vi "fill_sens_dat.vi"(6 "f_temp":T5 format="%_4g", 7 "rh_0":T1 caption="Relative Humidity (%)" format="%#_4g", 9 "raw_dat":string, 10 "index":i32, 11 "element in":T2={"states"=enum."idle", "bytes read"=0, "Response"="", "wr_buffr"="", "bytes_at_port"=0, "temp_clstr"={"sen_4_num"=0.0, "sen_3_num"=0.0, "sen_2_num"=0.0, "sen_1_num"=0.0, "sen_8_num"=0.0, "sen_7_num"=0.0, "sen_6_num"=0.0, "sen_5_num"=0.0, "dts"="", "sen_4"="", "sen_3"="", "sen_2"="", "sen_1"="", "sen_8"="", "sen_7"="", "sen_6"="", "sen_5"="", "temp_f_arry"=[], "sens_dat_raw_arry"=[], "raw_dat"="", "rh_arry"=[], "rh_1"=0.0, "rh_0"=0.0, "rh_3"=0.0, "rh_2"=0.0, "rh_5"=0.0, "rh_4"=0.0, "rh_7"=0.0, "rh_6"=0.0}, "logTable in"=[[["", "", "", "", "", "", "", "", "", ""], ["", "", "", "", "", "", "", "", "", ""], ["", "", "", "", "", "", "", "", "", ""], ["", "", "", "", "", "", "", "", "", ""], ["", "", "", "", "", "", "", "", "", ""], ["", "", "", "", "", "", "", "", "", ""], ["", "", "", "", "", "", "", "", "", " "]]], "mult_list"=0, "log_tabl_row_cnt"=0, "above_row_7"=FALSE, "sens_type"=0, "sens_type_arry"=[], "pibs_clstr"={"sens_typ_str"="", "rh_1"=0.0, "sen_8"="", "sen_7"="", "sen_6"="", "sen_5"="", "sen_4"="", "sen_3"="", "sen_2"="", "sen_1_num"=0.0, "sen_1"="", "rh_2"=0.0, "rh_3"=0.0, "sen_2_num"=0.0, "sen_3_num"=0.0, "sen_4_num"=0.0, "rh_4"=0.0, "sen_5_num"=0.0, "rh_5"=0.0, "sen_6_num"=0.0, "rh_6"=0.0, "sen_7_num"=0.0, "rh_7"=0.0, "sen_8_num"=0.0, "rh_8"=0.0, "sens_type_1"=0, "sens_type_2"=0, "sens_type_3"=0, "sens_type_4"=0, "sens_type_5"=0, "sens_type_6"=0, "sens_type_7"=0, "sens_type_8"=0, "sens_typ_str _2"=""}, "dts"=""} {"pibs_clstr"."sens_type_8" items=["SHTC3", "SHT3X", "D6T_1A", "HTS221", "AHT20", "ADT7410"]; "pibs_clstr"."sens_type_7" items=["SHTC3", "SHT3X", "D6T_1A", "HTS221", "AHT20", "ADT7410"]; "pibs_clstr"."sens_type_6" items=["SHTC3", "SHT3X", "D6T_1A", "HTS221", "AHT20", "ADT7410"]; "pibs_clstr"."sens_type_5" items=["SHTC3", "SHT3X", "D6T_1A", "HTS221", "AHT20", "ADT7410"]; "pibs_clstr"."sens_type_4" items=["SHTC3", "SHT3X", "D6T_1A", "HTS221", "AHT20", "ADT7410"]; "pibs_clstr"."sens_type_3" items=["SHTC3", "SHT3X", "D6T_1A", "HTS221", "AHT20", "ADT7410"]; "pibs_clstr"."sens_type_2" items=["SHTC3", "SHT3X", "D6T_1A", "HTS221", "AHT20", "ADT7410"]; "pibs_clstr"."sens_type_1" items=["SHTC3", "SHT3X", "D6T_1A", "HTS221", "AHT20", "ADT7410"]; "pibs_clstr"."rh_8" format="%#_4g"; "pibs_clstr"."sen_8_num" format="%_4g"; "pibs_clstr"."rh_7" format="%#_4g"; "pibs_clstr"."sen_7_num" format="%_4g"; "pibs_clstr"."rh_6" format="%#_4g"; "pibs_clstr"."sen_6_num" format="%_4g"; "pibs_clstr"."rh_5" format="%#_4g"; "pibs_clstr"."sen_5_num" format="%_4g"; "pibs_clstr"."rh_4" format="%#_4g"; "pibs_clstr"."sen_4_num" format="%_4g"; "pibs_clstr"."sen_3_num" format="%_4g"; "pibs_clstr"."sen_2_num" format="%_4g"; "pibs_clstr"."rh_3" format="%#_4g"; "pibs_clstr"."rh_2" format="%#_4g"; "pibs_clstr"."sen_1_num" format="%_4g"; "pibs_clstr"."rh_1" format="%#_4g"; "sens_type_arry" items=["SHTC3", "SHT3X", "D6T_1A", "HTS221", "AHT20", "ADT7410"]; "sens_type" items=["SHTC3", "SHT3X", "D6T_1A", "HTS221", "AHT20", "ADT7410"]; "temp_clstr"."rh_6" format="%#_4g"; "temp_clstr"."rh_7" format="%#_4g"; "temp_clstr"."rh_4" format="%#_4g"; "temp_clstr"."rh_5" format="%#_4g"; "temp_clstr"."rh_2" format="%#_4g"; "temp_clstr"."rh_3" format="%#_4g"; "temp_clstr"."rh_0" format="%#_4g"; "temp_clstr"."rh_1" format="%#_4g"; "temp_clstr"."rh_arry" format="%#_4g"; "temp_clstr"."temp_f_arry" format="%_4g"; "temp_clstr"."sen_5_num" format="%_4g"; "temp_clstr"."sen_6_num" format="%_4g"; "temp_clstr"."sen_7_num" format="%_4g"; "temp_clstr"."sen_8_num" format="%_4g"; "temp_clstr"."sen_1_num" format="%_4g"; "temp_clstr"."sen_2_num" format="%_4g"; "temp_clstr"."sen_3_num" format="%_4g"; "temp_clstr"."sen_4_num" format="%_4g"}) -> (3 "element out":T2={"states"=enum."idle", "bytes read"=0, "Response"="", "wr_buffr"="", "bytes_at_port"=0, "temp_clstr"={"sen_4_num"=0.0, "sen_3_num"=0.0, "sen_2_num"=0.0, "sen_1_num"=0.0, "sen_8_num"=0.0, "sen_7_num"=0.0, "sen_6_num"=0.0, "sen_5_num"=0.0, "dts"="", "sen_4"="", "sen_3"="", "sen_2"="", "sen_1"="", "sen_8"="", "sen_7"="", "sen_6"="", "sen_5"="", "temp_f_arry"=[], "sens_dat_raw_arry"=[], "raw_dat"="", "rh_arry"=[], "rh_1"=0.0, "rh_0"=0.0, "rh_3"=0.0, "rh_2"=0.0, "rh_5"=0.0, "rh_4"=0.0, "rh_7"=0.0, "rh_6"=0.0}, "logTable in"=[[["", "", "", "", "", "", "", "", "", ""], ["", "", "", "", "", "", "", "", "", ""], ["", "", "", "", "", "", "", "", "", ""], ["", "", "", "", "", "", "", "", "", ""], ["", "", "", "", "", "", "", "", "", ""], ["", "", "", "", "", "", "", "", "", ""], ["", "", "", "", "", "", "", "", "", " "]]], "mult_list"=0, "log_tabl_row_cnt"=0, "above_row_7"=FALSE, "sens_type"=0, "sens_type_arry"=[], "pibs_clstr"={"sens_typ_str"="", "rh_1"=0.0, "sen_8"="", "sen_7"="", "sen_6"="", "sen_5"="", "sen_4"="", "sen_3"="", "sen_2"="", "sen_1_num"=0.0, "sen_1"="", "rh_2"=0.0, "rh_3"=0.0, "sen_2_num"=0.0, "sen_3_num"=0.0, "sen_4_num"=0.0, "rh_4"=0.0, "sen_5_num"=0.0, "rh_5"=0.0, "sen_6_num"=0.0, "rh_6"=0.0, "sen_7_num"=0.0, "rh_7"=0.0, "sen_8_num"=0.0, "rh_8"=0.0, "sens_type_1"=0, "sens_type_2"=0, "sens_type_3"=0, "sens_type_4"=0, "sens_type_5"=0, "sens_type_6"=0, "sens_type_7"=0, "sens_type_8"=0, "sens_typ_str _2"=""}, "dts"=""} {"pibs_clstr"."sens_type_8" items=["SHTC3", "SHT3X", "D6T_1A", "HTS221", "AHT20", "ADT7410"]; "pibs_clstr"."sens_type_7" items=["SHTC3", "SHT3X", "D6T_1A", "HTS221", "AHT20", "ADT7410"]; "pibs_clstr"."sens_type_6" items=["SHTC3", "SHT3X", "D6T_1A", "HTS221", "AHT20", "ADT7410"]; "pibs_clstr"."sens_type_5" items=["SHTC3", "SHT3X", "D6T_1A", "HTS221", "AHT20", "ADT7410"]; "pibs_clstr"."sens_type_4" items=["SHTC3", "SHT3X", "D6T_1A", "HTS221", "AHT20", "ADT7410"]; "pibs_clstr"."sens_type_3" items=["SHTC3", "SHT3X", "D6T_1A", "HTS221", "AHT20", "ADT7410"]; "pibs_clstr"."sens_type_2" items=["SHTC3", "SHT3X", "D6T_1A", "HTS221", "AHT20", "ADT7410"]; "pibs_clstr"."sens_type_1" items=["SHTC3", "SHT3X", "D6T_1A", "HTS221", "AHT20", "ADT7410"]; "pibs_clstr"."rh_8" format="%#_4g"; "pibs_clstr"."sen_8_num" format="%_4g"; "pibs_clstr"."rh_7" format="%#_4g"; "pibs_clstr"."sen_7_num" format="%_4g"; "pibs_clstr"."rh_6" format="%#_4g"; "pibs_clstr"."sen_6_num" format="%_4g"; "pibs_clstr"."rh_5" format="%#_4g"; "pibs_clstr"."sen_5_num" format="%_4g"; "pibs_clstr"."rh_4" format="%#_4g"; "pibs_clstr"."sen_4_num" format="%_4g"; "pibs_clstr"."sen_3_num" format="%_4g"; "pibs_clstr"."sen_2_num" format="%_4g"; "pibs_clstr"."rh_3" format="%#_4g"; "pibs_clstr"."rh_2" format="%#_4g"; "pibs_clstr"."sen_1_num" format="%_4g"; "pibs_clstr"."rh_1" format="%#_4g"; "sens_type_arry" items=["SHTC3", "SHT3X", "D6T_1A", "HTS221", "AHT20", "ADT7410"]; "sens_type" items=["SHTC3", "SHT3X", "D6T_1A", "HTS221", "AHT20", "ADT7410"]; "temp_clstr"."rh_6" format="%#_4g"; "temp_clstr"."rh_7" format="%#_4g"; "temp_clstr"."rh_4" format="%#_4g"; "temp_clstr"."rh_5" format="%#_4g"; "temp_clstr"."rh_2" format="%#_4g"; "temp_clstr"."rh_3" format="%#_4g"; "temp_clstr"."rh_0" format="%#_4g"; "temp_clstr"."rh_1" format="%#_4g"; "temp_clstr"."rh_arry" format="%#_4g"; "temp_clstr"."temp_f_arry" format="%_4g"; "temp_clstr"."sen_5_num" format="%_4g"; "temp_clstr"."sen_6_num" format="%_4g"; "temp_clstr"."sen_7_num" format="%_4g"; "temp_clstr"."sen_8_num" format="%_4g"; "temp_clstr"."sen_1_num" format="%_4g"; "temp_clstr"."sen_2_num" format="%_4g"; "temp_clstr"."sen_3_num" format="%_4g"; "temp_clstr"."sen_4_num" format="%_4g"})   [LabVIEW 2013]
uses:
  temp_ind.ctl
  event_clstr.ctl
  states_cntrl.ctl
  log_dat.ctl
  rh_ind_arry.ctl
  rh_ind.ctl
  sens_type.ctl
  sens_type_arry_cntrl.ctl
  pibs_clstr.ctl
  sens_type_arry_str_cntrl.ctl
  raw_dat_str.ctl
  dts_cntrl.ctl
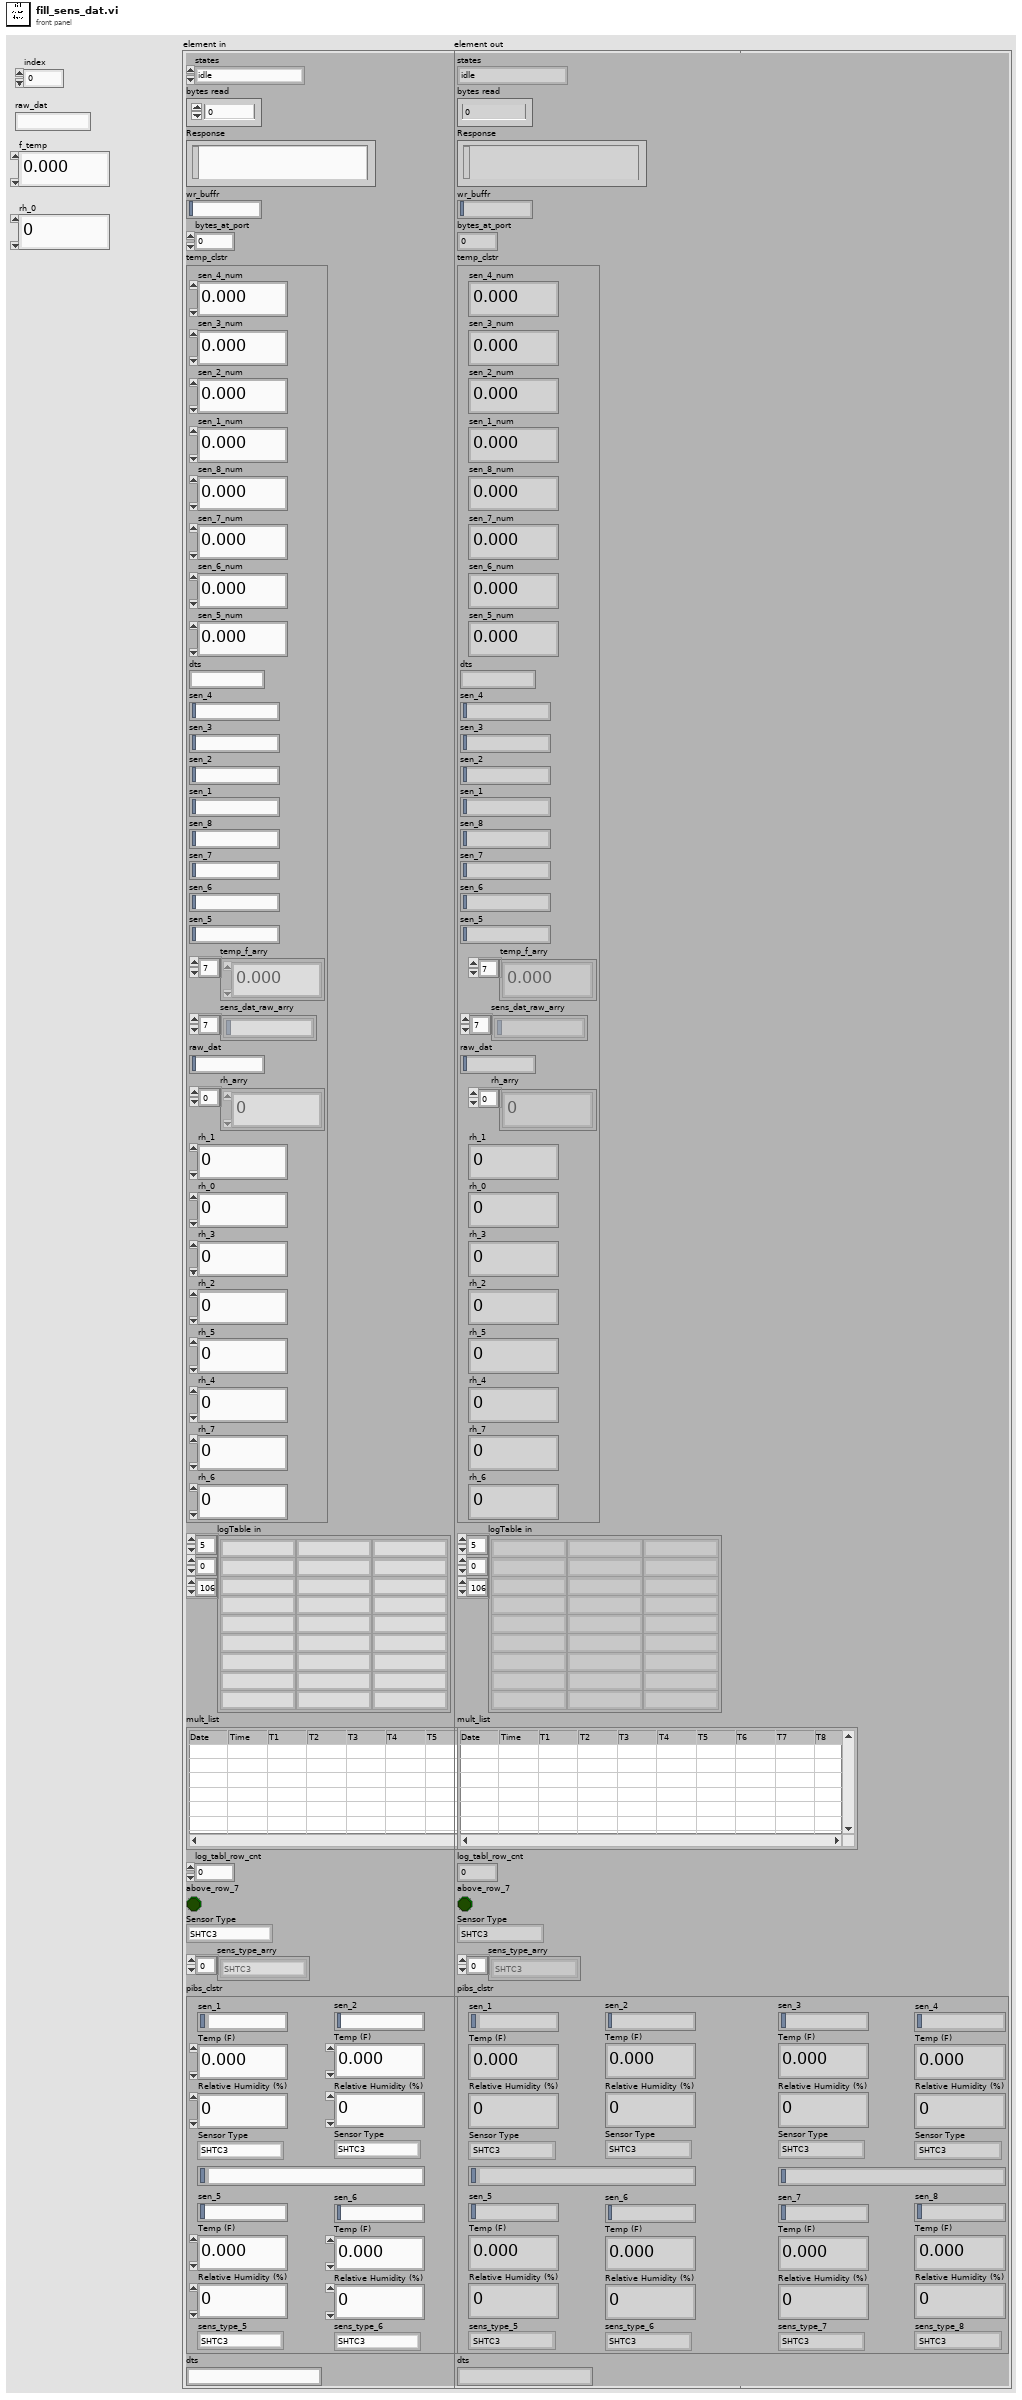
[diagram p1: front panel]
types:
  T1 = typedef "rh_ind.ctl" = dbl
  T2 = typedef "event_clstr.ctl" = cluster{"states":T3, "bytes read":u32, "Response":string, "wr_buffr":string, "bytes_at_port":u32, "temp_clstr":T4, "logTable in":string[][][], "mult_list":i32, "log_tabl_row_cnt":u64, "above_row_7":bool, "sens_type":T7, "sens_type_arry":T8, "pibs_clstr":T9, "dts":T12}
  T3 = typedef "states_cntrl.ctl" = enum16{"idle", "exit", "init", "obtain_q", "capt_data", "snd_sens_type", "send_cmd", "capt_wait", "read_data", "chk_bytes_rd", "disp_data", "sav_qry", "sav_dat", "dwell", "small_dwell", "stop_capt_qry", "go_to_minor_qsm", "retr_data"}
  T4 = typedef "log_dat.ctl" = cluster{"sen_4_num":T5, "sen_3_num":T5, "sen_2_num":T5, "sen_1_num":T5, "sen_8_num":T5, "sen_7_num":T5, "sen_6_num":T5, "sen_5_num":T5, "dts":string, "sen_4":string, "sen_3":string, "sen_2":string, "sen_1":string, "sen_8":string, "sen_7":string, "sen_6":string, "sen_5":string, "temp_f_arry":T5[], "sens_dat_raw_arry":string[], "raw_dat":string, "rh_arry":T6, "rh_1":T1, "rh_0":T1, "rh_3":T1, "rh_2":T1, "rh_5":T1, "rh_4":T1, "rh_7":T1, "rh_6":T1}
  T5 = typedef "temp_ind.ctl" = dbl
  T6 = typedef "rh_ind_arry.ctl" = T1[]
  T7 = typedef "sens_type.ctl" = u8
  T8 = typedef "sens_type_arry_cntrl.ctl" = T7[]
  T9 = typedef "pibs_clstr.ctl" = cluster{"sens_typ_str":T10, "rh_1":T1, "sen_8":T11, "sen_7":T11, "sen_6":T11, "sen_5":T11, "sen_4":T11, "sen_3":T11, "sen_2":T11, "sen_1_num":T5, "sen_1":T11, "rh_2":T1, "rh_3":T1, "sen_2_num":T5, "sen_3_num":T5, "sen_4_num":T5, "rh_4":T1, "sen_5_num":T5, "rh_5":T1, "sen_6_num":T5, "rh_6":T1, "sen_7_num":T5, "rh_7":T1, "sen_8_num":T5, "rh_8":T1, "sens_type_1":T7, "sens_type_2":T7, "sens_type_3":T7, "sens_type_4":T7, "sens_type_5":T7, "sens_type_6":T7, "sens_type_7":T7, "sens_type_8":T7, "sens_typ_str _2":T10}
  T10 = typedef "sens_type_arry_str_cntrl.ctl" = string
  T11 = typedef "raw_dat_str.ctl" = string
  T12 = typedef "dts_cntrl.ctl" = string
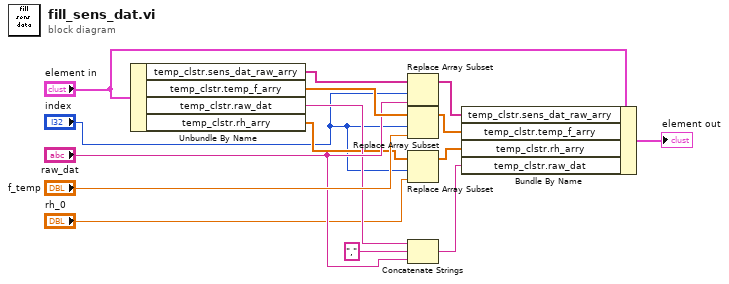
[diagram p0: block diagram]
diagram:
  n1 = Unbundle By Name("element in") -> ("temp_clstr.sens_dat_raw_arry"=w11:string[], "temp_clstr.temp_f_arry"=w10:T5[], "temp_clstr.raw_dat"=w6:string, "temp_clstr.rh_arry"=w4:T6)
  n2 = Replace Array Subset(array=w11, new element="raw_dat", index="index") -> (w12:string[])
  n3 = Replace Array Subset(array=w10, new element="f_temp", index="index") -> (w13:T5[])
  n4 = Replace Array Subset(array=w4, new element="rh_0", index="index") -> (w1:T6)
  n5 = Concatenate Strings(w6, "," ("string"), "raw_dat") -> (w5:string)
  n6 = Bundle By Name(cluster="element in", "temp_clstr.sens_dat_raw_arry"=w12, "temp_clstr.temp_f_arry"=w13, "temp_clstr.rh_arry"=w1, "temp_clstr.raw_dat"=w5) -> (→"element out":T2)
